vi "Set Waypoint Transfer Status.vi"(8 "Error In":errorcluster, 11 "Waypoint Transfer Status In":T1) -> (0 "Error Out":errorcluster)   [LabVIEW 2014]
uses:
  Controls/Waypoint Transfer Status.ctl
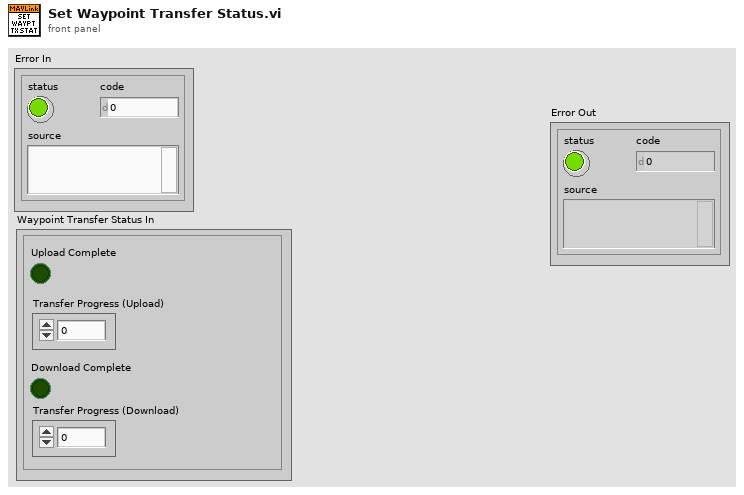
[diagram p1: front panel]
types:
  T1 = typedef "Waypoint Transfer Status.ctl" = cluster{"Upload Complete":bool, "Transfer Progress (Upload)":dbl, "Download Complete":bool, "Transfer Progress (Download)":dbl}
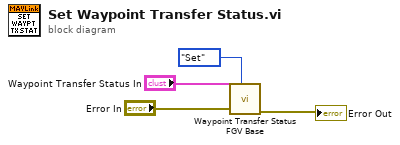
[diagram p0: block diagram]
diagram:
  n1 = call "Waypoint Transfer Status FGV Base.vi"("Method"=enum16{"Get", "Set"}."Set", "Error In"="Error In", "Status In"="Waypoint Transfer Status In") -> ("Error Out"=→"Error Out":errorcluster)  [unwired: 7 in, 1 out]
